vi "VI-Create KObject From Typedef.vi"() -> ()   [LabVIEW 2015]
uses:
  Controls/KTable/KTable.xctl
  Common SubVIs/VI-Typedef Table Element.ctl
panel:
  in  "Table":u16(xcontrol)
  out "exit":bool
  in  "NewClass":T1={"Folder"=path "D:/Experiment VIs", "Name"="New Class", "Typedef"=path "D:/Experiment VIs/Koop/KObject Class/KObject.lvclass"}
  in  "Create Class":bool
  # "KObject"
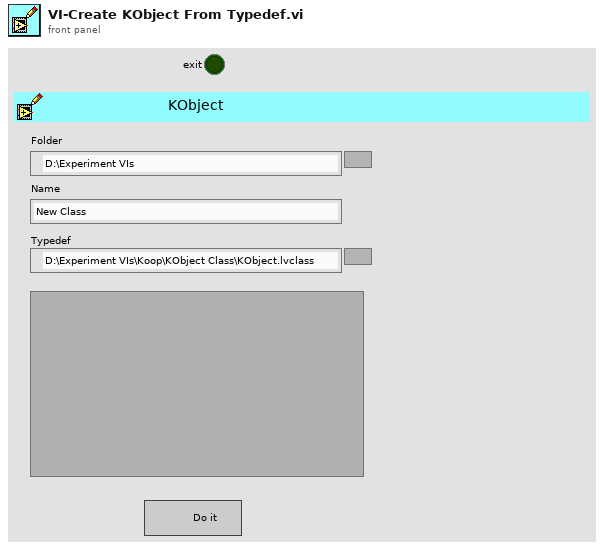
[diagram p1: front panel]
types:
  T1 = cluster{"Folder":path, "Name":string, "Typedef":path}
  T2 = typedef "VI-Typedef Table Element.ctl" = cluster{"Name":string, "Type":string, "Status":string}
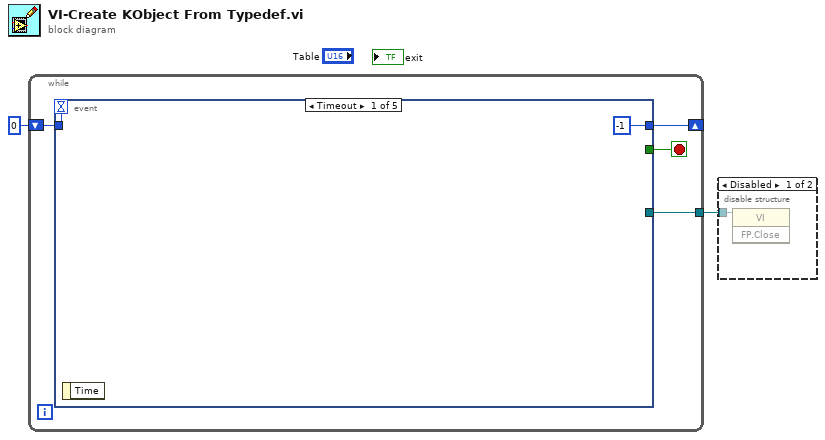
[diagram p0: block diagram]
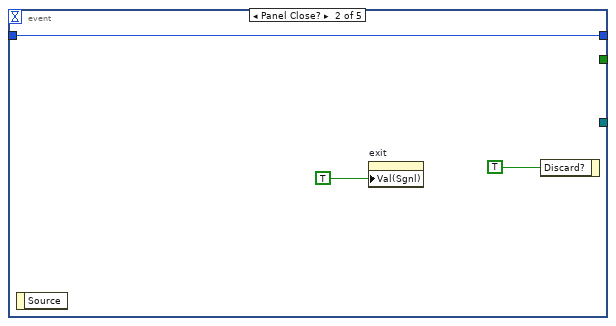
[diagram p3: hidden frame]
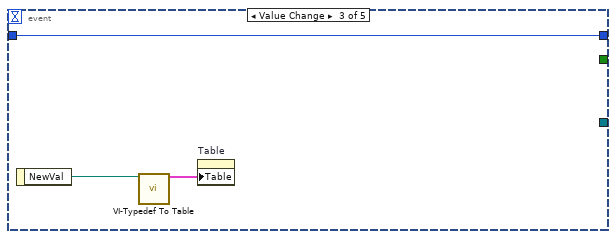
[diagram p4: hidden frame]
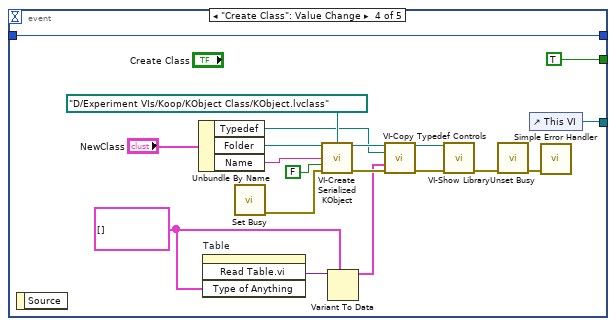
[diagram p5: hidden frame]
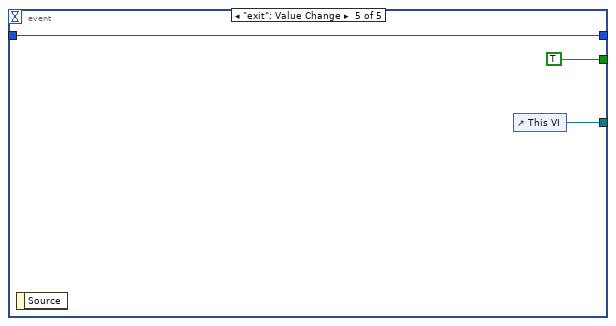
[diagram p6: hidden frame]
diagram:
  n1 = while {
    tunnel: [w6] -> w2
    shift-right: [w3] -> _
    shift-left: 0 -> [w4]
    stop <- w5 stop-if-true
    n2 = event shown="[0] Timeout" {
      selector: _ -> [_ _ _ _ _]
      dyn-events: _ -> [_ _ _ _ _]
      timeout: w4 -> [_ _ _ _ _]
      tunnel: [_ _ _ w30 w35] -> w6
      tunnel: [_ _ _ TRUE TRUE] -> w5
      tunnel: w4 -> [_ w8 w13 w28 w33]
      tunnel: [-1 w8 w13 w28 w33] -> w3
      event Timeout {
        n3 = event-data() -> ()  [unwired: 1 in, 1 out]
      }
      event Panel Close? {
        n4 = event-data() -> ()  [unwired: 1 in, 1 out]
        n5 = property on="exit" class="Bool (strict)"("Val(Sgnl)"=TRUE ("Value (Signaling)")) -> ()  [unwired: 2 in, 2 out]
        n6 = event-data("Discard?"=TRUE) -> ()  [unwired: 1 in, 1 out]
      }
      event "NewClass.Typedef": Value Change {
        n7 = event-data() -> ("NewVal"=w12:path)  [unwired: 1 in]
        n8 = call "VI-Typedef To Table.vi"("Path to typdef"=w12) -> ("Table"=w11:T2[])  [unwired: 13 in, 1 out]
        n9 = property on="Table" class="KTable (strict)"("Table"=w11) -> ()  [unwired: 2 in, 2 out]
      }
      event "Create Class": Value Change {
        w16 = T2[] [] ("Table")
        n10 = event-data() -> ()  [unwired: 1 in, 1 out]
        n11 = Unbundle By Name("NewClass") -> ("Typedef"=w18:path, "Folder"=w27:path, "Name"=w29:string)
        n12 = invoke on="Table" class="KTable (strict)" method="Read Table.vi"("Type of Anything"=w16) -> ("Read Table.vi"=w17:variant)  [unwired: 3 in, 3 out]
        n13 = call <vilib>:"Set Busy.vi"() -> ("error out"=w26:errorcluster)  [unwired: 10 in, 1 out]
        n14 = call "VI-Create Serialized KObject.vi"("Folder"=w27, "Base class path"=path "D:/Experiment VIs/Koop/KObject Class/KObject.lvclass", "Name"=w29, "Make base"=FALSE, "error in (no error)"=w26) -> ("Library"=w21:path, "error out"=w19:errorcluster)  [unwired: 9 in]
        n15 = Variant To Data(type=w16, Variant=w17) -> (data=w15:T2[])  [unwired: 1 in, 1 out]
        n16 = call "VI-Copy Typedef Controls.vi"("Library in"=w21, "Typedef"=w18, "Table"=w15, "error in (no error)"=w19) -> ("Library out"=w22:path, "error out"=w20:errorcluster)  [unwired: 10 in]
        n17 = call "VI-Show Library.vi"("Library Path"=w22, "error in (no error)"=w20) -> ("error out"=w23:errorcluster)  [unwired: 13 in]
        n18 = call <vilib>:"Unset Busy.vi"("error in (no error)"=w23) -> ("error out"=w25:errorcluster)  [unwired: 10 in]
        n19 = control-ref of="This VI"() -> (w30:refnum<vi>)
        n20 = call <vilib>:"Simple Error Handler.vi"("error in (no error)"=w25) -> ()  [unwired: 4 in, 5 out]
      }
      event "exit": Value Change {
        n21 = event-data() -> ()  [unwired: 1 in, 1 out]
        n22 = control-ref of="This VI"() -> (w35:refnum<vi>)
      }
    }
  }
  n23 = disable-structure shown="Disabled" {
    disable-tunnel: w2 -> [w36 _]
    frame Disabled {
      n24 = invoke class="VI" method="FP.Close"(reference=w36) -> ()  [unwired: 2 in, 3 out]
    }
    frame Enabled {
    }
  }
